vi "Write connection ID.vi"(8 "error in (no error)":errorcluster, 10 "connection ID":refnum<k24>, 11 "KinesisCube in":refnum<class "KinesisCube.lvclass">) -> (0 "error out":errorcluster, 3 "KinesisCube out":refnum<class "KinesisCube.lvclass">)   [LabVIEW 2020, in "KinesisCube.lvclass"]
uses:
  KinesisCube.lvclass
  C:/GEECS/Developers Version/source/Device Drivers/KinesisCube/Thorlabs.MotionControl.KCube.PiezoCLI.dll
  Thorlabs.MotionControl.KCube.PiezoCLI.dll
  KinesisCube.lvclass/KinesisCube.ctl
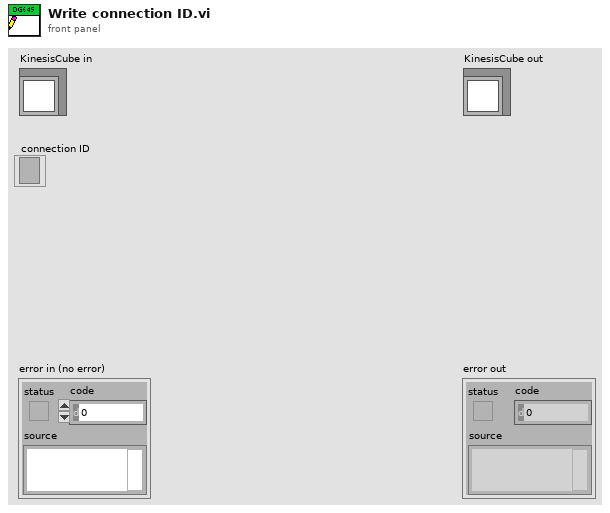
[diagram p1: front panel]
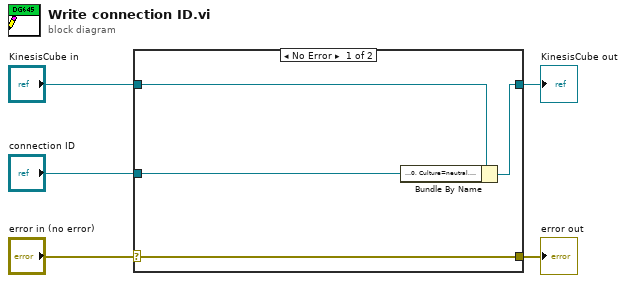
[diagram p0: block diagram]
diagram:
  n1 = case shown="No Error" "error in (no error)" {
    selector: "error in (no error)" -> [w9 w10]
    tunnel: [w9 w10] -> w4
    tunnel: [w7 w11] -> w2
    tunnel: "KinesisCube in" -> [w8 w11]
    tunnel: "connection ID" -> [w6 _]
    frame No Error {
      n2 = Bundle By Name(cluster=w8, "connection ID"=w6) -> (w7:refnum<class "KinesisCube.lvclass">)
    }
    frame Error {
    }
  }
  "error out" <- w4
  "KinesisCube out" <- w2
